vi "Send message (SubVI).vi"(0 "Exchange.lvclass":refnum<class "Exchange.lvclass">, 1 "target":string, 2 "Channel in":refnum<class "Channel.lvclass">, 3 "error in (no error)":errorcluster, 4 "body":string, 9 "Correlation ID":string) -> (5 "Exchange out":refnum<class "Exchange.lvclass">, 6 "Correlation ID out":string, 7 "Reply queue out":refnum<class "Queue.lvclass">, 8 "error out":errorcluster)   [LabVIEW 2016]
uses:
  <vilib>/Distrio/LabbitMQ/Exchange/Exchange.lvclass
  <vilib>/Distrio/LabbitMQ/Channel/Channel.lvclass
  <vilib>/Distrio/LabbitMQ/Queue/Queue.lvclass
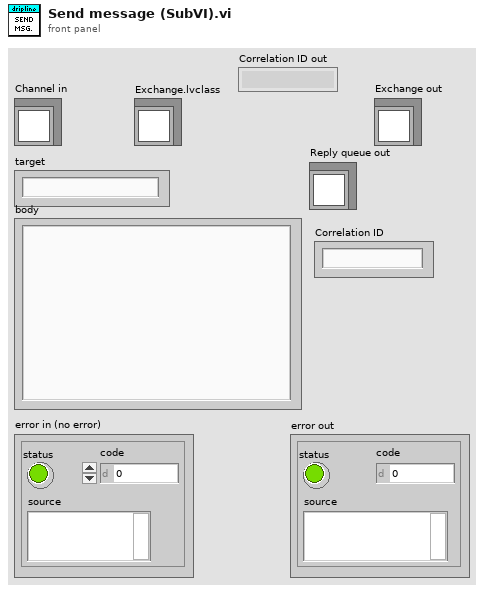
[diagram p1: front panel]
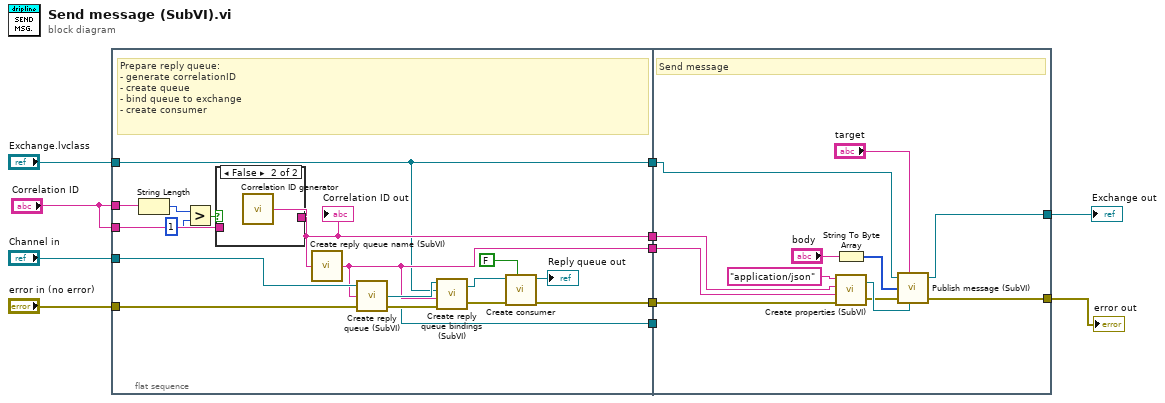
[diagram p0: block diagram]
diagram:
  n1 = flat-sequence {
    tunnel: "error in (no error)" -> [w29]
    tunnel: "Channel in" -> [w28]
    tunnel: "Exchange.lvclass" -> [w17]
    tunnel: [w21] -> w8
    tunnel: [w20] -> w7
    tunnel: [w19] -> w6
    tunnel: [w18] -> w5
    tunnel: [w17] -> w4
    tunnel: "Correlation ID" -> [w16]
    tunnel: "Correlation ID" -> [w14]
    tunnel: w8 -> [w43]
    tunnel: w7 -> [_]
    tunnel: w6 -> [w41]
    tunnel: w5 -> [w40]
    tunnel: w4 -> [w34]
    tunnel: [w33] -> w3
    tunnel: [w32] -> w2
    frame #0 {
      # "Prepare reply queue:\n- generate correlationID\n- create queue\n- bind queue to exchange\n- create consumer"
      n2 = String Length(string=w16) -> (length=w15:i32)
      n3 = Greater?(x=w15, y=1) -> (0:w13:bool)
      n4 = case shown="False" w13 {
        tunnel: [w30 w31] -> w18
        tunnel: w14 -> [w30 _]
        frame True {
        }
        frame False {
          n5 = call "Correlation ID generator.vi"() -> ("Correlation ID"=w31:string)  [unwired: 1 in]
        }
      }
      "Correlation ID out" <- w18
      n6 = call "Create reply queue name (SubVI).vi"("Correlation ID"=w18) -> ("reply queue name"=w19:string)
      n7 = call "Create reply queue (SubVI).vi"("error in (no error)"=w29, "queue name"=w19, "Channel in"=w28) -> ("error out"=w26:errorcluster, "Queue.lvclass"=w27:refnum<class "Queue.lvclass">, "Channel out"=w20:refnum<class "Channel.lvclass">)
      n8 = call "Create reply queue bindings (SubVI).vi"("error in (no error)"=w26, "reply queue name"=w19, "Exchange.lvclass"=w17, "Queue in"=w27) -> ("error out"=w25:errorcluster, "Queue out"=w24:refnum<class "Queue.lvclass">)
      n9 = call <vilib>:"Create consumer.vi"("noAck? (T)"=FALSE, "error in (no error)"=w25, "Queue in"=w24) -> ("error out"=w21:errorcluster, "Queue out"=→"Reply queue out":refnum<class "Queue.lvclass">)  [unwired: 7 in]
    }
    frame #1 {
      # "Send message"
      n10 = String To Byte Array(string="body") -> (unsigned byte array=w38:u8[])
      n11 = call "Create properties (SubVI).vi"("error in (no error)"=w43, "ReplyTo"=w41, "CorrelationId"=w40, "ContentEncoding"="application/json") -> ("error out"=w36:errorcluster, "reference out"=w37:refnum<k24>)
      n12 = call "Publish message (SubVI).vi"("Exchange in"=w34, "target"="target", "body"=w38, "error in (no error)"=w36, "MessageProperties"=w37) -> ("Exchange out"=w32:refnum<class "Exchange.lvclass">, "error out"=w33:errorcluster)  [unwired: 1 in]
    }
  }
  "error out" <- w3
  "Exchange out" <- w2
